vi "Part 1.vi"(11 "Input":string) -> (3 "Output":i64)   [LabVIEW 2021]
uses:
  6ace44e6-f576-493f-8eb8-f58c948b0551.vi
  <userlib>/_OpenG.lib/string/string.llb/Convert EOLs (String)__ogtk.vi
  <vilib>/Comparison/Equal/Equal Functor/Equal Functor.lvclass
panel:
  out "array":string[](array[string])
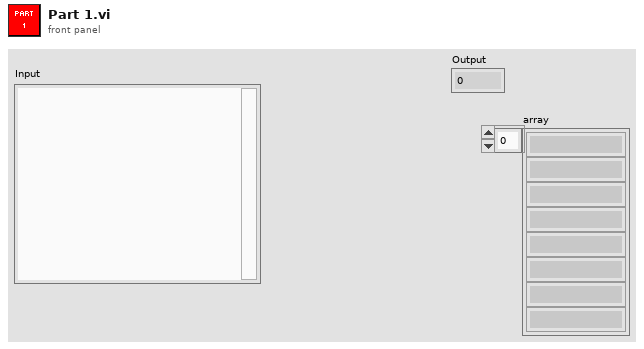
[diagram p1: front panel]
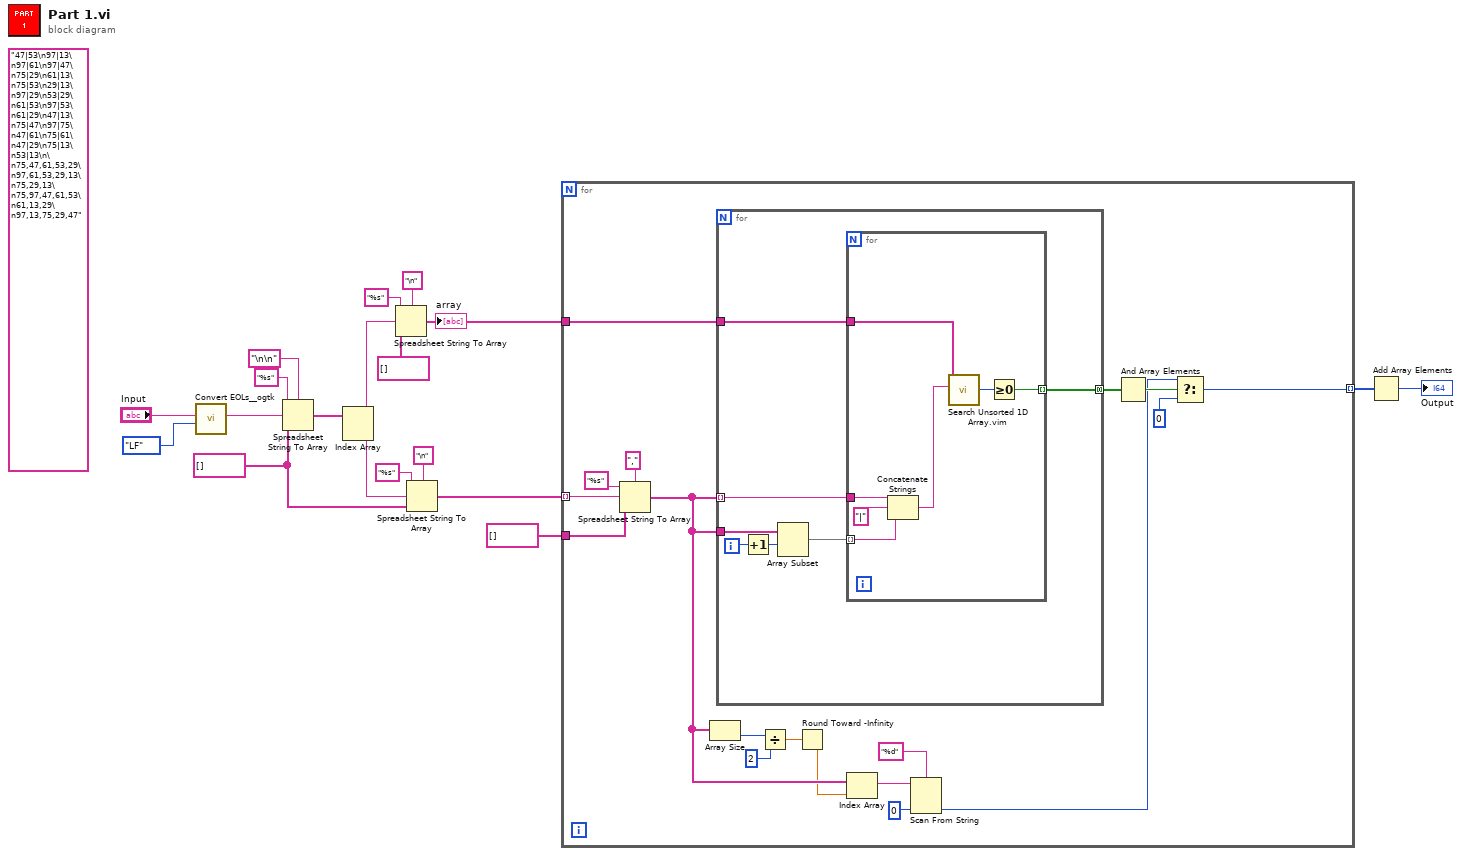
[diagram p0: block diagram]
diagram:
  (unwired) "47|53\n97|13\n97|61\n97|47\n75|29\n61|13\n75|53\n29|13\n97|29\n53|29\n61|53\n97|53\n61|29\n47|13\n75|47\n97|75\n47|61\n75|61\n47|29\n75|13\n53|13\n\n75,47,61,53,29\n97,61,53,29,13\n75,29,13\n75,97,47,61,53\n61,13,29\n97,13,75,29,47"
  w13 = string[] []
  n1 = call-poly <userlib>:"Convert EOLs__ogtk.vi"("Convert to:"=enum16{"CR", "LF", "CRLF"}."LF", "String in"="Input") -> ("String out"=w17:string)  [unwired: 9 in]
  n2 = Spreadsheet String To Array(delimiter (Tab)="\n\n", format string="%s", spreadsheet string=w17, array type (2D Dbl)=w13) -> (array=w15:string[])
  n3 = Index Array(array=w15) -> (element #1=w6:string, element #2=w14:string)  [unwired: 2 in]
  n4 = Spreadsheet String To Array(delimiter (Tab)="\n", format string="%s", spreadsheet string=w6, array type (2D Dbl)=string[] []) -> (array=w4:string[])
  "array" <- w4
  n5 = Spreadsheet String To Array(delimiter (Tab)="\n", format string="%s", spreadsheet string=w14, array type (2D Dbl)=w13) -> (array=w10:string[])
  n6 = for {
    tunnel: w10 -> [w37] mode=indexing
    tunnel: string[] [] -> [w36]
    tunnel: w4 -> [w33]
    tunnel: [w29] -> w3 mode=indexing
    n7 = Spreadsheet String To Array(delimiter (Tab)=",", format string="%s", spreadsheet string=w37, array type (2D Dbl)=w36) -> (array=w25:string[])
    n8 = Array Size(array=w25) -> (size(s)=w28:i32)
    n9 = for {
      tunnel: w25 -> [w40] mode=indexing
      tunnel: w25 -> [w44]
      tunnel: w33 -> [w39]
      tunnel: [w38] -> w32 mode=concatenating
      i -> [w43]
      n10 = Increment(x=w43) -> (x+1=w42:i32)
      n11 = Array Subset(array=w44, index=w42) -> (w41:string[])  [unwired: 1 in]
      n12 = for {
        tunnel: w41 -> [w50] mode=indexing
        tunnel: w40 -> [w51]
        tunnel: w39 -> [w48]
        tunnel: [w45] -> w38 mode=indexing
        n13 = Concatenate Strings(w51, "|", w50) -> (w47:string)
        n14 = call "Search Unsorted 1D Array.vim"("element"=w47, "unsorted 1D array"=w48) -> ("index of element"=w46:i32)  [unwired: 9 in]
        n15 = Greater Or Equal To 0?(x=w46) -> (x >= 0?=w45:bool)
      }
    }
    n16 = Divide(x=w28, y=2) -> (x/y=w26:dbl)
    n17 = Round Toward -Infinity(1:w26) -> (0:w24:dbl)
    n18 = Index Array(array=w25, index=w24) -> (element=w23:string)
    n19 = Scan From String(format string="%d", input string=w23, default 1=i64 0) -> (output 1=w20:i64)  [unwired: 2 in, 3 out]
    n20 = And Array Elements(Boolean array=w32) -> (logical AND=w31:bool)
    n21 = Select(t=w20, s=w31, f=i64 0) -> (s? t:f=w29:i64)
  }
  n22 = Add Array Elements(numeric array=w3) -> (sum=→"Output":i64)
